vi "控件大小手柄.vi"() -> ()   [LabVIEW 2010]
panel:
  out "量表":dbl(knob) scale=0.0..10.0
  in  "确定按钮":bool
  in  "数值":dbl
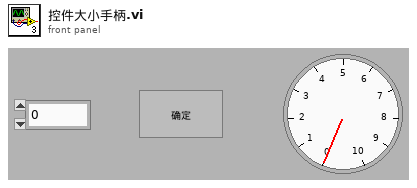
[diagram p1: front panel]
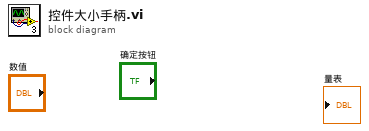
[diagram p0: block diagram]
diagram:
